vi "binary_get_array.vi"(8 "error in":errorcluster, 11 "path to binary file":path) -> (0 "error out":errorcluster, 3 "binary data":u8[](array[numeric]))   [LabVIEW 2017]
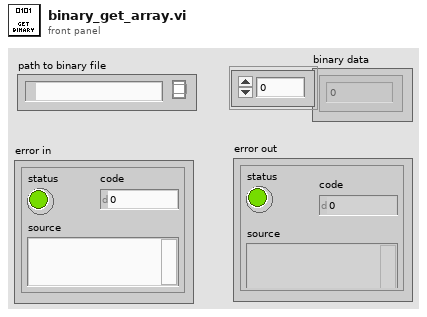
[diagram p1: front panel]
types:
  T1 = enum16{"big-endian, network order", "native, host order", "little-endian"}
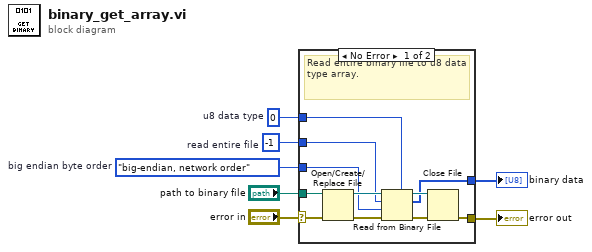
[diagram p0: block diagram]
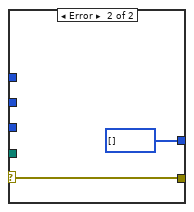
[diagram p2: hidden frame]
diagram:
  w4 = u8 0  # u8 data type
  w5 = -1  # read entire file
  w6 = T1."big-endian, network order"  # big endian byte order
  n1 = case shown="No Error" "error in" {
    selector: "error in" -> [w9 w20]
    tunnel: "path to binary file" -> [w16 _]
    tunnel: w6 -> [w15 _]
    tunnel: w5 -> [w12 _]
    tunnel: w4 -> [w11 _]
    tunnel: [w8 w20] -> w2
    tunnel: [w10 u8[] [] ("defaultValue")] -> w1
    frame No Error {
      # "Read entire binary file to u8 data type array."
      n2 = Open/Create/Replace File(file path (use dialog)=w16, error in=w9) -> (refnum out=w18:refnum<file>, error out=w13:errorcluster)  [unwired: 4 in, 1 out]
      n3 = Read from Binary File(5:w11, 8:w13, 9:w15, 10:w12, 11:w18) -> (0:w14:errorcluster, 2:w10:u8[], 3:w17:refnum<file>)  [unwired: 1 in, 1 out]
      n4 = Close File(refnum=w17, error in=w14) -> (error out=w8:errorcluster)  [unwired: 1 out]
    }
    frame Error {
    }
  }
  "error out" <- w2
  "binary data" <- w1
